vi "cluster-to-csv-format.vi"(9 "Sensors":T1 {"Temperature 3 (degC)" format="%0.2f"; "Temperature 2 (degC)" format="%0.2f"; "Temperature 1 (degC)" format="%0.2f"}, 11 "Time String":string) -> (3 "spreadsheet string":string)   [LabVIEW 2021]
uses:
  generic-sensor-logger/typedefs/sensor-values.ctl
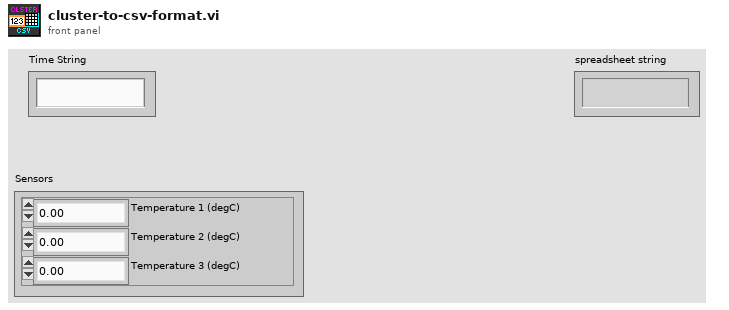
[diagram p1: front panel]
types:
  T1 = typedef "sensor-values.ctl" = cluster{"Temperature 1 (degC)":dbl, "Temperature 2 (degC)":dbl, "Temperature 3 (degC)":dbl}
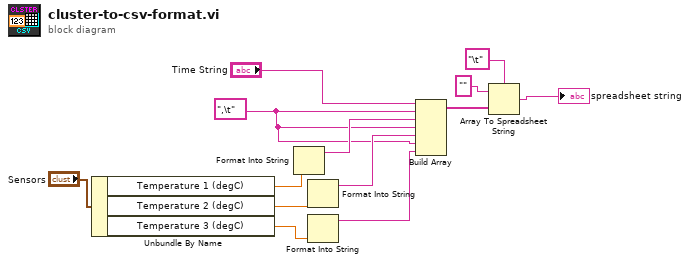
[diagram p0: block diagram]
diagram:
  w3 = ",\t" ("element")
  n1 = Unbundle By Name("Sensors") -> ("Temperature 1 (degC)"=w6:dbl, "Temperature 2 (degC)"=w5:dbl, "Temperature 3 (degC)"=w2:dbl)
  n2 = Format Into String(w6) -> (resulting string=w8:string)  [unwired: 3 in, 1 out]
  n3 = Format Into String(w5) -> (resulting string=w4:string)  [unwired: 3 in, 1 out]
  n4 = Format Into String(w2) -> (resulting string=w1:string)  [unwired: 3 in, 1 out]
  n5 = Build Array "Build Array"("Time String", w3, w8, w3, w4, w3, w1) -> (w10:string[])
  n6 = Array To Spreadsheet String(delimiter (Tab)="\t", array=w10, 3:"" ("format string")) -> (spreadsheet string=→"spreadsheet string":string)
